vi "DeCoF open TCP connection.vi"(4 "error in (no error)":errorcluster, 5 "TCP_NODELAY (true)":bool=TRUE, 6 "remote port":u16=1998, 7 "address":string) -> (0 "error out":errorcluster, 3 "TCP Connection ID":T1)   [LabVIEW 2013]
doc: "Opens a TCP/IP connection and set the TCP_NO_DELAY option."
uses:
  DeCoF connection.ctl
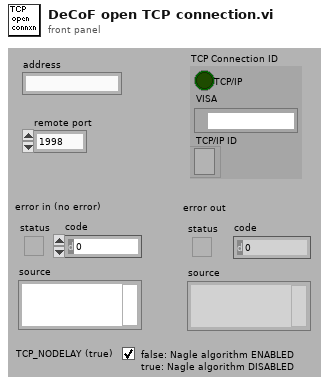
[diagram p1: front panel]
types:
  T1 = typedef "DeCoF connection.ctl" = cluster{"TCP/IP":bool, "VISA":refnum<visa-resource-name>, "TCP/IP ID":refnum<k5>}
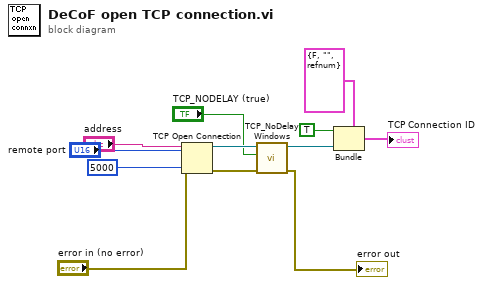
[diagram p0: block diagram]
diagram:
  n1 = TCP Open Connection(address="address", remote port or service name="remote port", timeout ms (60000)=5000, error in (no error)="error in (no error)") -> (connection ID=w7:refnum<k5>, error out=w9:errorcluster)  [unwired: 1 in]
  n2 = call "TCP_NoDelay Windows.vi"("error in (no error)"=w9, "TCP_NODELAY (true)"="TCP_NODELAY (true)", "connID"=w7) -> ("error out"=→"error out":errorcluster, "connID 2"=w4:refnum<k5>)  [unwired: 3 in]
  n3 = Bundle(cluster=T1 {"TCP/IP"=FALSE, "VISA"="", "TCP/IP ID"=refnum} ("TCP Connection ID"), "TCP/IP"=TRUE, "TCP/IP ID"=w4) -> (→"TCP Connection ID":T1)  [unwired: 1 in]
